vi "GetCANFrame.vi"(8 "error in (no error)":errorcluster, 11 "Variant":variant) -> (0 "error out":errorcluster, 2 "Valid?":bool, 3 "PathArrayToString":string)   [LabVIEW 2016, in "LIN Frame Protection Addon System Explorer.lvlib"]
uses:
  LIN Frame Protection Addon System Explorer.lvlib
  NationalInstruments.VeriStand
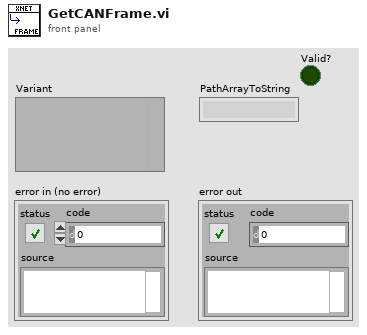
[diagram p1: front panel]
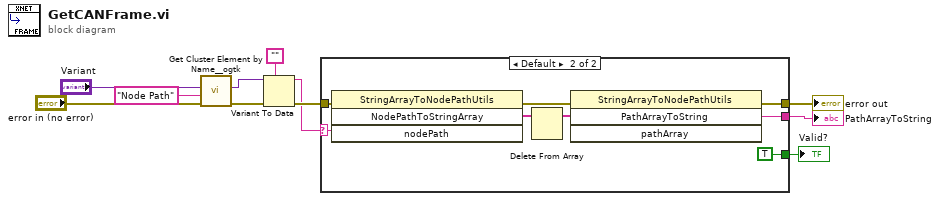
[diagram p0: block diagram]
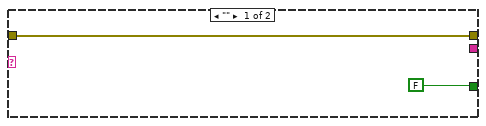
[diagram p2: hidden frame]
diagram:
  n1 = call <userlib>:"Get Cluster Element by Name__ogtk.vi"("error in (no error)"="error in (no error)", "Element Name"="Node Path", "Cluster"="Variant") -> ("error out"=w5:errorcluster, "VElement"=w6:variant)  [unwired: 6 in, 1 out]
  n2 = Variant To Data(error in=w5, type="", Variant=w6) -> (data=w3:string, error out=w9:errorcluster)
  n3 = case shown="Default" w3 {
    selector: w3 -> [_ w15]
    tunnel: [w13 w21] -> w10
    tunnel: w9 -> [w13 w19]
    tunnel: [_ w18] -> w2
    tunnel: [FALSE TRUE] -> w1
    frame "" {
    }
    frame Default {
      n4 = invoke class="StringArrayToNodePathUtils" method="NodePathToStringArray"(error in=w19, "nodePath"=w15) -> (error out=w20:errorcluster, "NodePathToStringArray"=w16:string[])  [unwired: 2 in, 2 out]
      n5 = Delete From Array(array=w16) -> (array with subset deleted=w17:string[])  [unwired: 2 in, 1 out]
      n6 = invoke class="StringArrayToNodePathUtils" method="PathArrayToString"(error in=w20, "pathArray"=w17) -> (error out=w21:errorcluster, "PathArrayToString"=w18:string)  [unwired: 2 in, 2 out]
    }
  }
  "error out" <- w10
  "PathArrayToString" <- w2
  "Valid?" <- w1
